vi "DSF.Engine.Transceiver.Command.Send.vi"(8 "error in (no error)":errorcluster, 9 "timeout in ms (0)":i32 format="%d ms", 10 "command":T1, 11 "Transceiver Thread in":refnum<class "DSF.Engine.Transceiver Thread.lvclass">) -> (0 "error out":errorcluster, 1 "timed out?":bool, 3 "Transceiver Thread out":refnum<class "DSF.Engine.Transceiver Thread.lvclass">)   [LabVIEW 2017, in "DSF.Engine.lvlib" / "DSF.Engine.Transceiver Thread.lvclass"]
uses:
  DSF.Engine.Transceiver Thread.lvclass
  Plugin/DSF.Engine.Plugin.lvclass
  Interface/DSF.Engine.Interface.Transceiver.lvclass
  Interface/DSF.Engine.Interface.Transceiver.Write.Command.vi
  Interface/DSF.Engine.Interface.Transceiver.Command.ctl
  Interface/DSF.Engine.Interface.Transceiver.Command Data.ctl
  Interface/DSF.Engine.Interface.Transceiver.Command Parameters.ctl
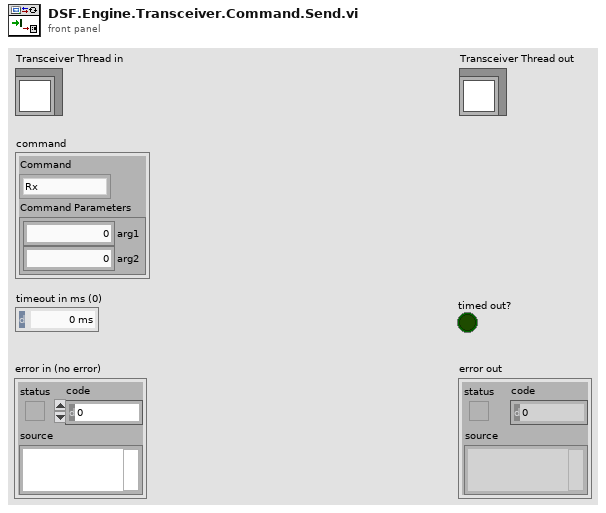
[diagram p1: front panel]
types:
  T1 = typedef "DSF.Engine.lvlib/DSF.Engine.Interface.Transceiver.lvclass/DSF.Engine.Interface.Transceiver.Command Data.ctl" = cluster{"Command":T2, "Command Parameters":T3}
  T2 = typedef "DSF.Engine.lvlib/DSF.Engine.Interface.Transceiver.lvclass/DSF.Engine.Interface.Transceiver.Command.ctl" = enum8{"Rx", "Tx", "Shutdown"}
  T3 = typedef "DSF.Engine.lvlib/DSF.Engine.Interface.Transceiver.lvclass/DSF.Engine.Interface.Transceiver.Command Parameters.ctl" = cluster{"arg1":u64, "arg2":u64}
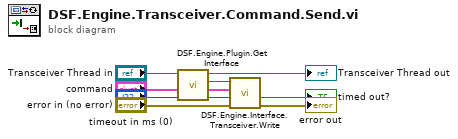
[diagram p0: block diagram]
diagram:
  n1 = call "DSF.Engine.Plugin.Get Interface.vi"("Plugin in"="Transceiver Thread in") -> ("Interface"=w7:refnum<class "DSF.Engine.Interface.Transceiver.lvclass">, "Plugin out"=→"Transceiver Thread out":refnum<class "DSF.Engine.Plugin.lvclass">)  [unwired: 9 in]
  n2 = call-poly "DSF.Engine.Interface.Transceiver.Write.vi"("error in (no error)"="error in (no error)", "timeout in ms (0)"="timeout in ms (0)", "command"="command", "Transceiver Interface in"=w7) -> ("error out"=→"error out":errorcluster, "timed out?"=→"timed out?":bool)  [unwired: 5 in, 1 out]
